vi "Select Point File FGV Operation.vi"(7 "Oper.":T1, 8 "error in":errorcluster) -> (0 "error out":errorcluster)   [LabVIEW 2016]
uses:
  Select Point File FGV Operation.ctl
panel:
  in  "FilePath":path
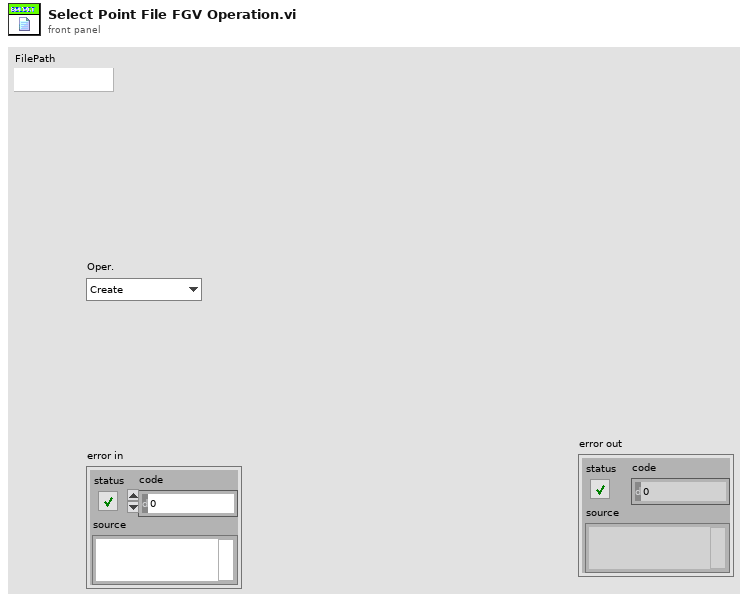
[diagram p1: front panel]
types:
  T1 = typedef "Select Point File FGV Operation.ctl" = enum16{"Create", "Write", "Close"}
  T2 = typedef "Select Point Mode.ctl" = i32
  T3 = cluster{"Interval(s)":i32, "SavePara.SelectPointMode":T2, "FilePath":path, "FileHead":string, "CHName(Unit)":string[], "CHName":string[], "CHUnit":string[], "TemplatePath":path}
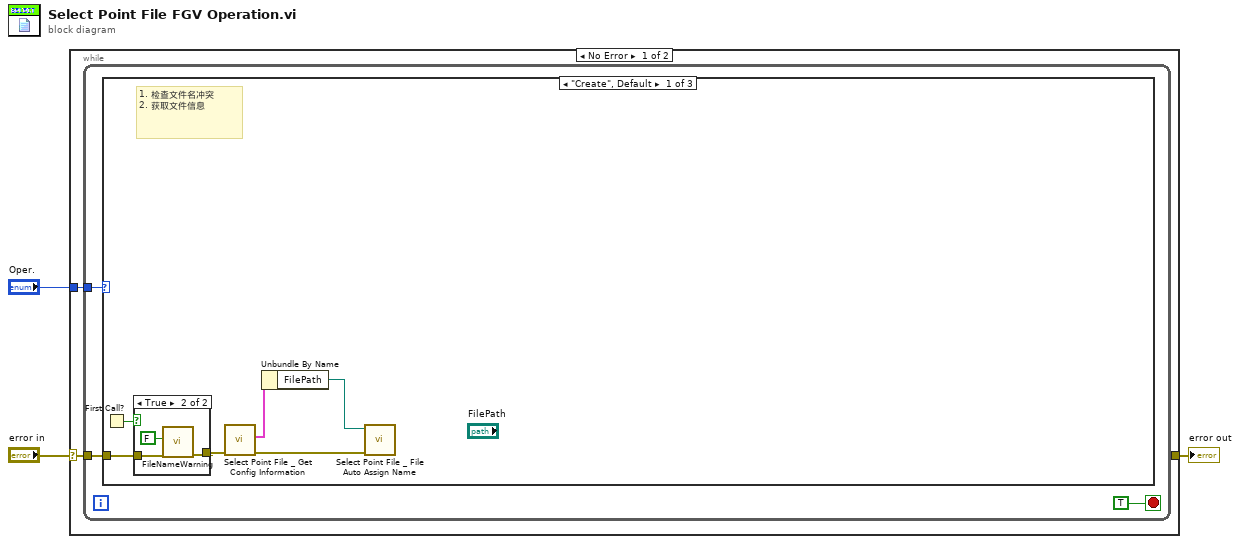
[diagram p0: block diagram]
diagram:
  n1 = case shown="No Error" "error in" {
    selector: "error in" -> [w4 w19]
    tunnel: "Oper." -> [w5 _]
    tunnel: [_ w19] -> w1
    frame No Error {
      n2 = while {
        tunnel: w5 -> [w8]
        tunnel: w4 -> [w6]
        stop <- TRUE stop-if-true
        n3 = case shown="\"Create\", Default" w8 {
          tunnel: w6 -> [w12 _ _]
          frame "Create", Default {
            # "1. 检查文件名冲突 \n2. 获取文件信息"
            n4 = First Call?() -> (First Call?: T/F=w13:bool)
            n5 = case shown="True" w13 {
              tunnel: w12 -> [w15 w18]
              tunnel: [w15 w17] -> w11
              frame False {
              }
              frame True {
                n6 = call "FileNameWarning.vi"("error in"=w18, "ContinuousFile？"=FALSE) -> ("error out"=w17:errorcluster)  [unwired: 9 in]
              }
            }
            n7 = call "Select Point File _ Get Config Information.vi"("error in"=w11) -> ("error out"=w10:errorcluster, "Info"=w14:T3)  [unwired: 9 in]
            n8 = Unbundle By Name(w14) -> ("FilePath"=w9:path)
            n9 = call "Select Point File _ File Auto Assign Name.vi"("error in"=w10, "FilePathIn"=w9) -> ()  [unwired: 8 in, 2 out]
          }
          frame "Write" {
          }
          frame "Close" {
          }
        }
      }
    }
    frame Error {
    }
  }
  "error out" <- w1
